vi "ConfigInputLoopStart.vi"(1 "MulticolumnListbox in":refnum<vi>, 2 "ID":u8, 3 "ItemNames in":string[][](array[string])) -> (0 "ItemNames out":string[][](array[string]))   [LabVIEW 2018, in "Config.lvlib"]
uses:
  Config.lvlib
panel:
  in  "Replace":bool
  in  "Insert":bool
  in  "Append":bool
  in  "Iterations":u16=1 min=1 step=1
  # "Loop Start"
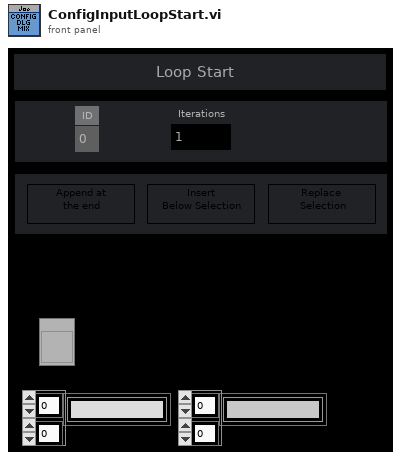
[diagram p1: front panel]
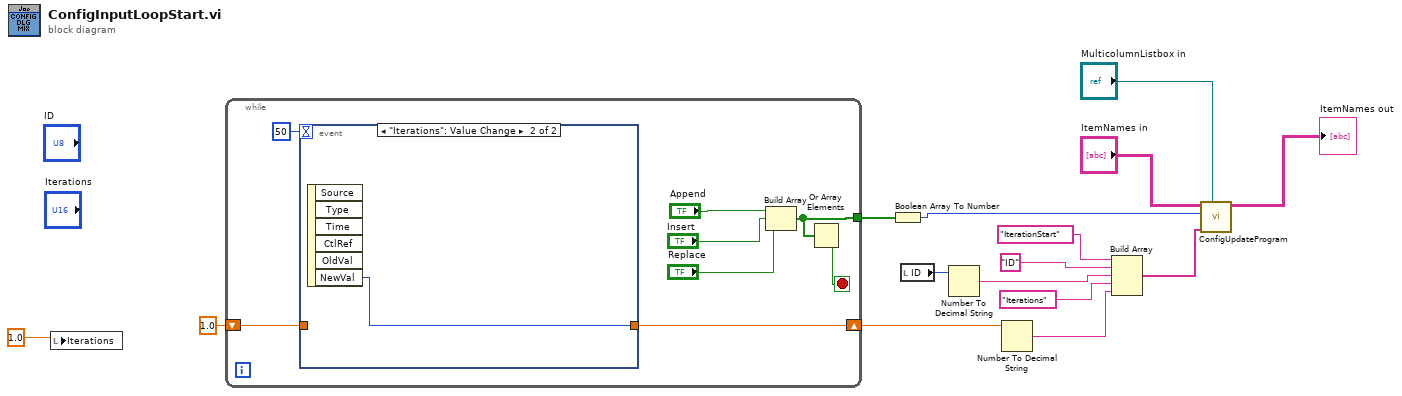
[diagram p0: block diagram]
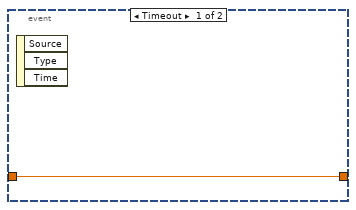
[diagram p2: hidden frame]
diagram:
  n1 = local write "Iterations"(1.0 ("Mixing Cycles")) -> ()
  n2 = while {
    tunnel: [w18] -> w14
    shift-right: [w17] -> w2
    shift-left: 1.0 ("NewVal") -> [w16]
    stop <- w19 stop-if-true
    n3 = event shown="[1] \"Iterations\": Value Change" {
      selector: _ -> [_ _]
      dyn-events: _ -> [_ _]
      timeout: 50 -> [_ _]
      tunnel: [w24 w25] -> w17
      tunnel: w16 -> [w24 _]
      event Timeout {
        n4 = event-data() -> ()  [unwired: 1 in, 3 out]
      }
      event "Iterations": Value Change {
        n5 = event-data() -> ("NewVal"=w25:u16)  [unwired: 1 in, 5 out]
      }
    }
    n6 = Build Array("Append", "Insert", "Replace") -> (w18:bool[])
    n7 = Or Array Elements(Boolean array=w18) -> (logical OR=w19:bool)
  }
  n8 = Boolean Array To Number(Boolean array=w14) -> (number=w12:u32)
  n9 = local read "ID"() -> (w1:u8)
  n10 = Number To Decimal String(number=w1) -> (decimal integer string=w7:string)  [unwired: 1 in]
  n11 = Number To Decimal String(number=w2) -> (decimal integer string=w4:string)  [unwired: 1 in]
  n12 = Build Array("IterationStart", "ID" ("element"), w7, "Iterations", w4) -> (w3:string[])
  n13 = call "ConfigUpdateProgram.vi"("MulticolumnListbox in"="MulticolumnListbox in", "New Element"=w3, "Operation"=w12, "ItemNames in"="ItemNames in") -> ("ItemNames out"=→"ItemNames out":string[][])  [unwired: 7 in]
